vi "Configure Sweep (Frequency-Power).vi"(0 "VISA resource name":refnum<visa-resource-name>, 1 "Stop/Span (100E-6 V)":dbl=0.0001 format="%^#_9g", 5 "Sweep Parameter (0: DC Control Voltage)":enum16{"DC Control Voltage", "DC Power Voltage"}(ring), 7 "Sweep Type (1: Center/Span)":enum16{"Start/Stop", "Center/Span"}(ring)=enum."Center/Span", 9 "Start/Center (50E-6 V)":dbl=5e-05 format="%^#_9g", 11 "error in (no error)":errorcluster) -> (4 "VISA resource name out":refnum<visa-resource-name>, 15 "error out":errorcluster)   [LabVIEW 2011, in "Agilent E5052X.lvlib"]
doc: "Sets the range in which measurements will be taken for the Frequency/Power measurement.\n\n<b>Note:</b>\n\n1) \"Configure Measurement Characteristics(Freq-Power)\" VI must be run before this VI."
uses:
  Agilent E5052X.lvlib
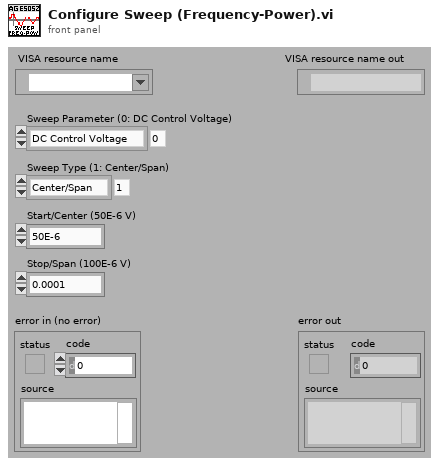
[diagram p1: front panel]
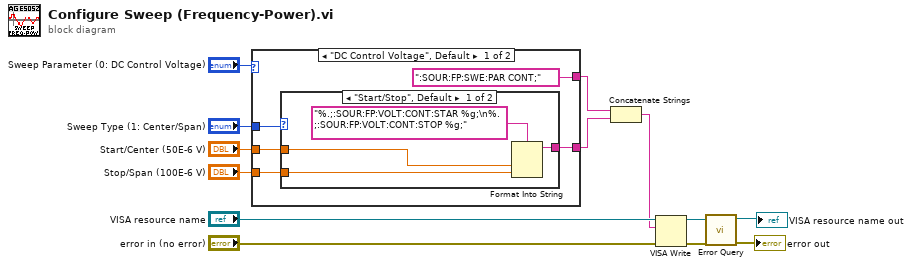
[diagram p0: block diagram]
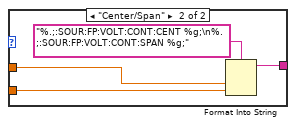
[diagram p2: hidden frame]
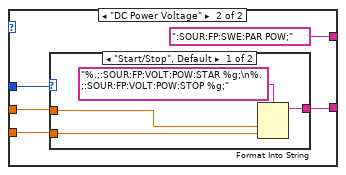
[diagram p3: hidden frame]
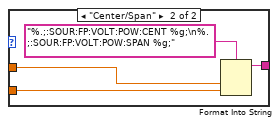
[diagram p4: hidden frame]
diagram:
  n1 = case shown="\"DC Control Voltage\", Default" "Sweep Parameter (0: DC Control Voltage)" {
    tunnel: [":SOUR:FP:SWE:PAR CONT;" ":SOUR:FP:SWE:PAR POW;"] -> w9
    tunnel: "Sweep Type (1: Center/Span)" -> [w18 w30]
    tunnel: "Start/Center (50E-6 V)" -> [w17 w29]
    tunnel: "Stop/Span (100E-6 V)" -> [w16 w28]
    tunnel: [w14 w27] -> w8
    frame "DC Control Voltage", Default {
      n2 = case shown="\"Start/Stop\", Default" w18 {
        tunnel: w17 -> [w21 w25]
        tunnel: w16 -> [w22 w24]
        tunnel: [w19 w23] -> w14
        frame "Start/Stop", Default {
          n3 = Format Into String(format string="%.;:SOUR:FP:VOLT:CONT:STAR %g;\n%.;:SOUR:FP:VOLT:CONT:STOP %g;", w21, w22) -> (resulting string=w19:string)  [unwired: 2 in, 1 out]
        }
        frame "Center/Span" {
          n4 = Format Into String(format string="%.;:SOUR:FP:VOLT:CONT:CENT %g;\n%.;:SOUR:FP:VOLT:CONT:SPAN %g;", w25, w24) -> (resulting string=w23:string)  [unwired: 2 in, 1 out]
        }
      }
    }
    frame "DC Power Voltage" {
      n5 = case shown="\"Start/Stop\", Default" w30 {
        tunnel: w29 -> [w34 w38]
        tunnel: w28 -> [w35 w37]
        tunnel: [w32 w36] -> w27
        frame "Start/Stop", Default {
          n6 = Format Into String(format string="%.;:SOUR:FP:VOLT:POW:STAR %g;\n%.;:SOUR:FP:VOLT:POW:STOP %g;", w34, w35) -> (resulting string=w32:string)  [unwired: 2 in, 1 out]
        }
        frame "Center/Span" {
          n7 = Format Into String(format string="%.;:SOUR:FP:VOLT:POW:CENT %g;\n%.;:SOUR:FP:VOLT:POW:SPAN %g;", w38, w37) -> (resulting string=w36:string)  [unwired: 2 in, 1 out]
        }
      }
    }
  }
  n8 = Concatenate Strings(w9, w8) -> (w5:string)
  n9 = VISA Write(VISA resource name="VISA resource name", write buffer=w5, error in (no error)="error in (no error)") -> (VISA resource name out=w4:refnum<visa-resource-name>, error out=w3:errorcluster)  [unwired: 1 out]
  n10 = call "Error Query.vi"("error in (no error)"=w3, "VISA resource name"=w4) -> ("error out"=→"error out":errorcluster, "VISA resource name out"=→"VISA resource name out":refnum<visa-resource-name>)  [unwired: 6 in, 2 out]
